vi "Auton Selector.vi"() -> ()   [LabVIEW 2017]
panel:
  out "3/LRL/Scale":bool
  out "3/RLR/Switch":bool
  out "3/LLL/Exist":bool
  out "3/RRR/Scale":bool
  out "3/RRR/Switch":bool
  out "2/All/Switch":bool
  out "1/LLL/Swich":bool
  in  "Scale":bool
  in  "Switch":bool
  out "1/LLL/Scale":bool
  out "1/LRL/Switch":bool
  out "1/RLR/Scale":bool
  out "1/RRR/Exist":bool
  in  "Position":dbl
  in  "Field State":string
  out "Switch":bool
  out "Scale":bool
  out "Exist":bool
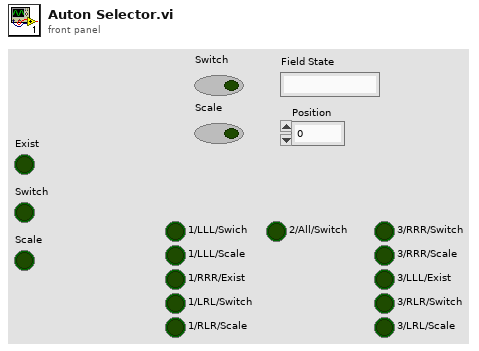
[diagram p1: front panel]
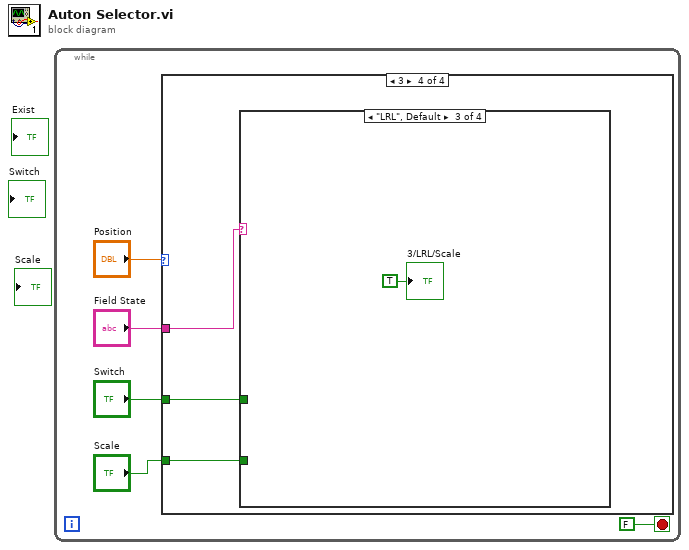
[diagram p0: block diagram]
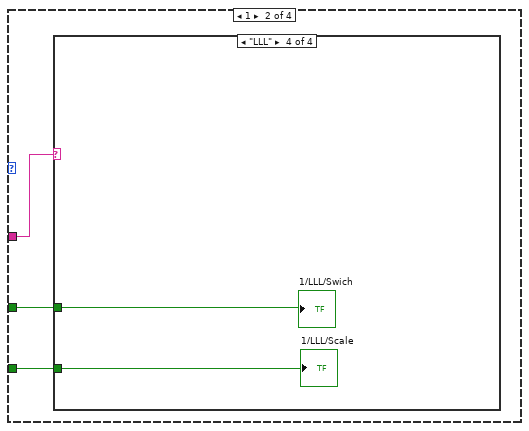
[diagram p3: hidden frame]
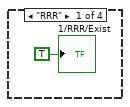
[diagram p4: hidden frame]
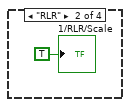
[diagram p5: hidden frame]
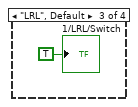
[diagram p6: hidden frame]
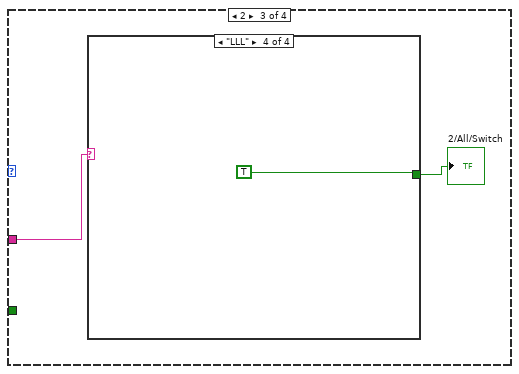
[diagram p7: hidden frame]
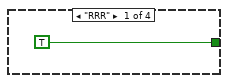
[diagram p8: hidden frame]
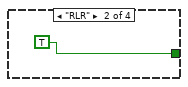
[diagram p9: hidden frame]
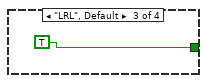
[diagram p10: hidden frame]
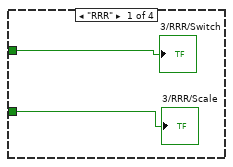
[diagram p11: hidden frame]
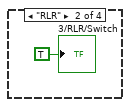
[diagram p12: hidden frame]
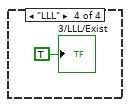
[diagram p13: hidden frame]
diagram:
  n1 = while {
    stop <- FALSE stop-if-true
    n2 = case shown="3" "Position" {
      tunnel: "Field State" -> [_ w8 w15 w22]
      tunnel: "Scale" -> [_ w7 _ w20]
      tunnel: "Switch" -> [_ w6 _ w21]
      frame 0, Default {
      }
      frame 1 {
        n3 = case shown="\"LLL\"" w8 {
          tunnel: w7 -> [_ _ _ w13]
          tunnel: w6 -> [_ _ _ w12]
          frame "RRR" {
            "1/RRR/Exist" <- TRUE ("Exist 2")
          }
          frame "RLR" {
            "1/RLR/Scale" <- TRUE ("Scale 2")
          }
          frame "LRL", Default {
            "1/LRL/Switch" <- TRUE ("Switch 2")
          }
          frame "LLL" {
            "1/LLL/Scale" <- w13
            "1/LLL/Swich" <- w12
          }
        }
      }
      frame 2 {
        n4 = case shown="\"LLL\"" w15 {
          tunnel: [TRUE TRUE TRUE TRUE] -> w14
          frame "RRR" {
          }
          frame "RLR" {
          }
          frame "LRL", Default {
          }
          frame "LLL" {
          }
        }
        "2/All/Switch" <- w14
      }
      frame 3 {
        n5 = case shown="\"LRL\", Default" w22 {
          tunnel: w21 -> [w24 _ _ _]
          tunnel: w20 -> [w23 _ _ _]
          frame "RRR" {
            "3/RRR/Switch" <- w24
            "3/RRR/Scale" <- w23
          }
          frame "RLR" {
            "3/RLR/Switch" <- TRUE ("Switch 2")
          }
          frame "LRL", Default {
            "3/LRL/Scale" <- TRUE ("Scale 2")
          }
          frame "LLL" {
            "3/LLL/Exist" <- TRUE ("Exist 2")
          }
        }
      }
    }
  }
